vi "ROI entry-Select whole plane.vi"() -> (0 "error IO":errorcluster)   [LabVIEW 2013]
uses:
  Typedefs/ROI management FG states.ctl
  Typedefs/ROI ID Enum.ctl
  <resource>/objmgr/IMAQImage.rc
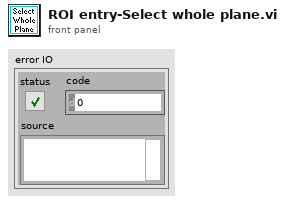
[diagram p1: front panel]
types:
  T1 = typedef "IMAQ Image.ctl" = refnum<image>
  T2 = typedef "ROI management FG states.ctl" = enum16{"Read", "Write", "Clear Last", "Clear All", "Update ROIs time", "Reload last ROI set", "Offset all ROI", "Offset visible ROI"}
  T3 = typedef "ROI ID Enum.ctl" = enum16{"Point", "MiniScan", "Comp. MiniScan", "Rectangle", "Comp. volume", "Arb. plane point"}
  T4 = typedef "ROI parameters data type.ctl" = cluster{"ROI index":dbl, "ROI ID":dbl, "ROI Time (ns)":dbl, "Pixels in ROI":dbl, "X start":dbl, "Y start":dbl, "Z start":dbl, "X stop":dbl, "Y stop":dbl, "Z stop":dbl, "Angle (deg)":dbl, "Composite ID":dbl, "Number of lines":dbl, "Frame Size":dbl, "Zoom":dbl, "Laser Power (%)":dbl, "ROI group ID":dbl}
  T5 = typedef "ROI spec.ctl" = cluster{"Coordinates":i32[], "Zoom":dbl, "ROI Enum":T3, "ZplaneIndex":i32}
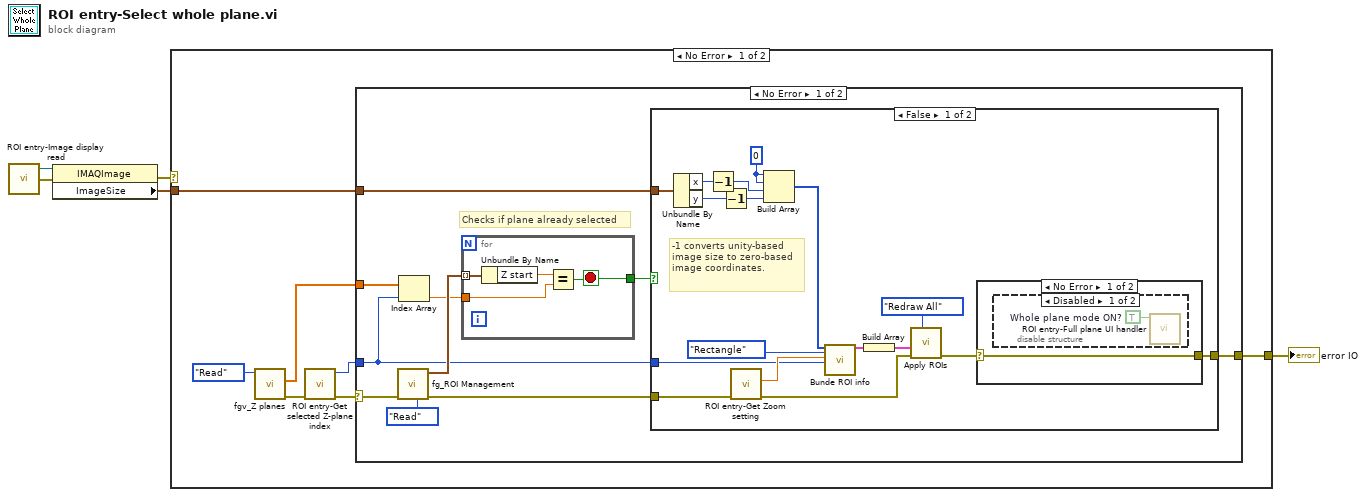
[diagram p0: block diagram]
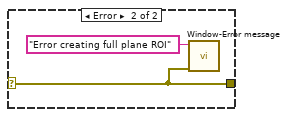
[diagram p3: hidden frame]
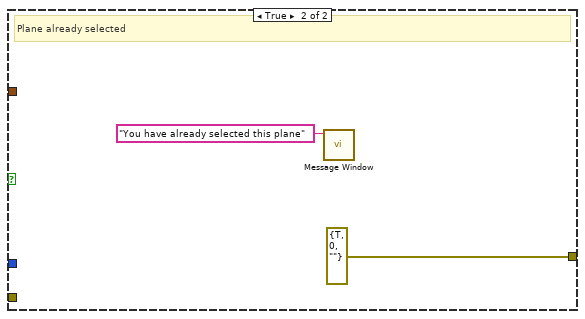
[diagram p4: hidden frame]
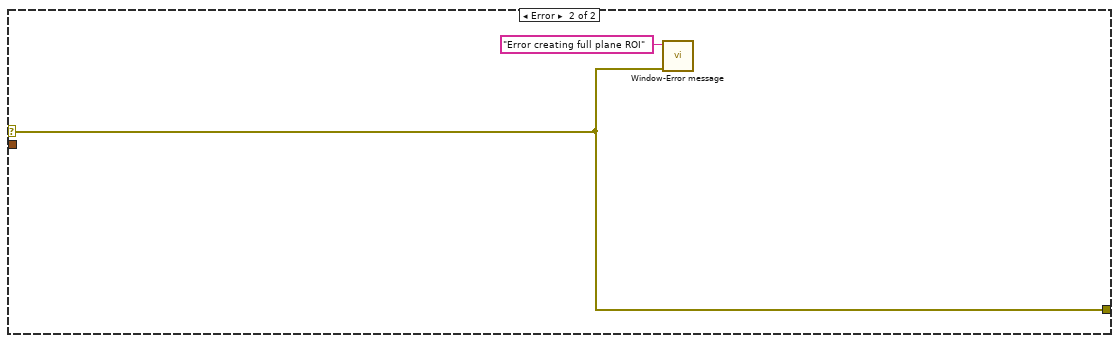
[diagram p6: hidden frame]
diagram:
  n1 = call "ROI entry-Image display read.vi"() -> ("error out"=w1:errorcluster, "CurrentImage"=w2:T1)  [unwired: 4 in]
  n2 = property class="IMAQImage"(reference=w2, error in=w1) -> (error out=w4:errorcluster, "ImageSize"=w5:cluster{"x":i32, "y":i32})  [unwired: 1 out]
  n3 = case shown="No Error" w4 {
    selector: w4 -> [_ w51]
    tunnel: w5 -> [w12 _]
    tunnel: [w11 w51] -> w3
    frame No Error {
      n4 = call "fgv_Z planes.vi"("Function"=enum16{"Intialize", "Write", "Read", "Clear"}."Read") -> ("error out"=w7:errorcluster, "AOL Z Planes"=w9:dbl[])  [unwired: 8 in, 1 out]
      n5 = call "ROI entry-Get selected Z-plane index.vi"("error in (no error)"=w7) -> ("error out"=w6:errorcluster, "Z-plane selector (index)"=w8:i32)  [unwired: 9 in]
      n6 = case shown="No Error" w6 {
        selector: w6 -> [w14 w50]
        tunnel: w12 -> [w18 _]
        tunnel: [w17 w50] -> w11
        tunnel: w9 -> [w16 _]
        tunnel: w8 -> [w15 _]
        frame No Error {
          # "Checks if plane already selected"
          n7 = call "fg_ROI Management.vi"("Function"=ROI_management_FG_states."Read", "error in (no error)"=w14) -> ("error out"=w13:errorcluster, "ROI Setup"=w21:T4[])  [unwired: 5 in, 3 out]
          n8 = Index Array(array=w16, index=w15) -> (element=w20:dbl)
          n9 = for {
            tunnel: w21 -> [w49] mode=indexing
            tunnel: w20 -> [w47]
            tunnel: [w46] -> w19
            stop <- w46 stop-if-true
            n10 = Unbundle By Name(w49) -> ("Z start"=w48:dbl)
            n11 = Equal?(x=w48, y=w47) -> (x = y?=w46:bool)
          }
          n12 = case shown="False" w19 {
            tunnel: w18 -> [w34 _]
            tunnel: w15 -> [w25 _]
            tunnel: [w32 errorcluster {"status"=TRUE, "code"=0, "source"=""} ("error IO")] -> w17
            tunnel: w13 -> [w29 _]
            frame False {
              w38 = 0
              # "-1 converts unity-based image size to zero-based image coordinates."
              n13 = Unbundle By Name(w34) -> ("x"=w36:i32, "y"=w35:i32)
              n14 = Decrement(x=w36) -> (x-1=w24:i32)
              n15 = Decrement(x=w35) -> (x-1=w23:i32)
              n16 = call "ROI entry-Get Zoom setting.vi"("error in (no error)"=w29) -> ("error out"=w30:errorcluster, "Zoom Value"=w31:dbl)  [unwired: 8 in, 1 out]
              n17 = Build Array(w38, w38, w24, w23) -> (w26:i32[])
              n18 = call "Bunde ROI info.vi"("ROI Coordinates"=w26, "ROI Enum"=ROI_ID_Enum."Rectangle", "Zoom"=w31, "ZplaneIndex"=w25) -> ("ROI Info"=w39:T5)  [unwired: 15 in]
              n19 = Build Array(w39) -> (w37:T5[])
              n20 = call "Apply ROIs.vi"("Mode (Redraw All)"=enum16{"Redraw All", "Draw Last"}."Redraw All", "error in (no error)"=w30, "ROIs Info []"=w37) -> ("error out"=w33:errorcluster)  [unwired: 5 in, 3 out]
              n21 = case shown="No Error" w33 {
                selector: w33 -> [w40 w42]
                tunnel: [w40 w42] -> w32
                frame No Error {
                  n22 = disable-structure shown="Disabled" {
                    frame Disabled {
                      w41 = TRUE  # Whole plane mode ON?
                      n23 = call "ROI entry-Full plane UI handler.vi"("Whole plane mode ON"=w41) -> ()  [unwired: 10 in, 1 out]
                    }
                    frame Enabled {
                    }
                  }
                }
                frame Error {
                  n24 = call "Window-Error message.vi"("error in (no error)"=w42, "Message"="Error creating full plane ROI") -> ()  [unwired: 9 in, 1 out]
                }
              }
            }
            frame True {
              # "Plane already selected"
              n25 = call "Message Window.vi"("Message string"="You have already selected this plane") -> ()  [unwired: 10 in, 1 out]
            }
          }
        }
        frame Error {
        }
      }
    }
    frame Error {
      n26 = call "Window-Error message.vi"("error in (no error)"=w51, "Message"="Error creating full plane ROI") -> ()  [unwired: 9 in, 1 out]
    }
  }
  "error IO" <- w3
